vi "Bin2.vi"(11 "Image Src":T1) -> (3 "Image":T1(plugin-control))   [LabVIEW 2011]
uses:
  <vilib>/vision/Image Controls.llb/IMAQ Image.ctl
  <vilib>/vision/NI_Vision_Development_Module.lvlib
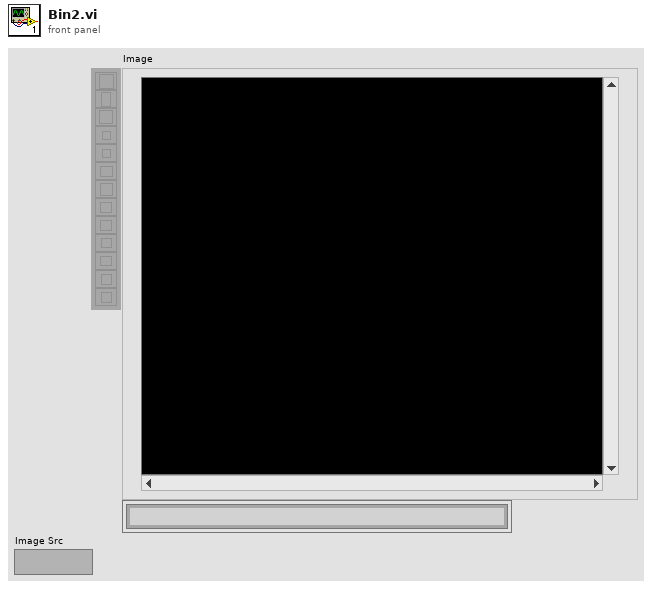
[diagram p1: front panel]
types:
  T1 = typedef "IMAQ Image.ctl" = refnum<image>
  T2 = typedef "Image Type" = u32
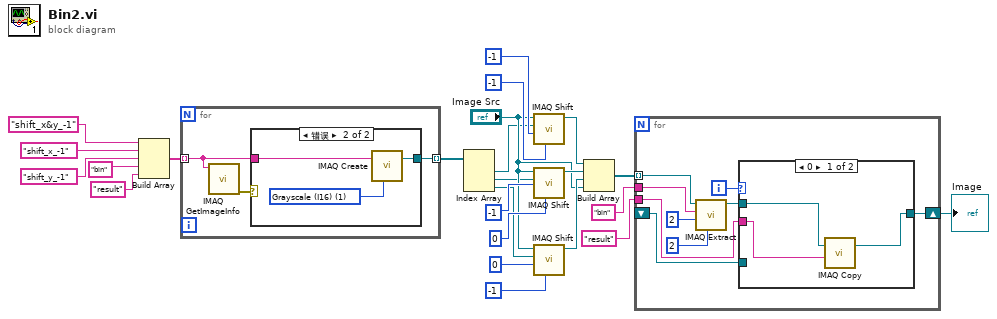
[diagram p0: block diagram]
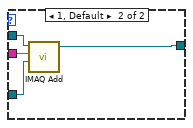
[diagram p3: hidden frame]
diagram:
  n1 = Build Array("shift_x&y_-1" ("Image Name"), "shift_x_-1" ("Image Name"), "shift_y_-1" ("Image Name"), "bin" ("Image Name"), "result" ("Image Name")) -> (w12:string[])
  n2 = for {
    tunnel: w12 -> [w26] mode=indexing
    tunnel: [w25] -> w8 mode=indexing
    n3 = call "IMAQ GetImageInfo"("Image"=w26) -> ("error out"=w27:errorcluster)  [unwired: 3 in, 7 out]
    n4 = case shown="错误" w27 {
      tunnel: w26 -> [w28 w30]
      tunnel: [w28 w29] -> w25
      frame No Error {
      }
      frame Error {
        w31 = T2 1 items=["Grayscale (U8)", "Grayscale (I16)", "Grayscale (SGL)", "Complex (CSG)", "RGB (U32)", "HSL (U32)", "RGB (U64)", "Grayscale (U16)"] ("Image Type")
        n5 = call "IMAQ Create"("Image Name"=w30, "Image Type"=w31) -> ("New Image"=w29:T1)  [unwired: 3 in, 1 out]
      }
    }
  }
  n6 = Index Array(array=w8) -> (element #1=w7:T1, element #2=w6:T1, element #3=w5:T1)  [unwired: 3 in]
  n7 = call "IMAQ Shift"("YOffset"=-1, "XOffset"=-1, "Image Dst"=w7, "Image Src"="Image Src") -> ("Image Dst Out"=w18:T1)  [unwired: 6 in, 1 out]
  n8 = call "IMAQ Shift"("YOffset"=0, "XOffset"=-1, "Image Dst"=w6, "Image Src"="Image Src") -> ("Image Dst Out"=w17:T1)  [unwired: 6 in, 1 out]
  n9 = call "IMAQ Shift"("YOffset"=-1, "XOffset"=0, "Image Dst"=w5, "Image Src"="Image Src") -> ("Image Dst Out"=w16:T1)  [unwired: 6 in, 1 out]
  n10 = Build Array(w18, w17, w16, "Image Src") -> (w15:T1[])
  n11 = for {
    tunnel: w15 -> [w37] mode=indexing
    shift-right: [w35] -> w14
    shift-left: _ -> [w34]
    tunnel: "bin" ("Image Name") -> [w33]
    tunnel: "result" ("Image Name") -> [w32]
    i -> [w40]
    n12 = call "IMAQ Extract"("Y Step Size"=2, "X Step Size"=2, "Image Dst"=w33, "Image Src"=w37) -> ("Image Dst Out"=w36:T1)  [unwired: 6 in, 1 out]
    n13 = case shown="0" w40 {
      tunnel: w36 -> [w43 w47]
      tunnel: [w41 w44] -> w35
      tunnel: w34 -> [_ w46]
      tunnel: w32 -> [w42 w45]
      frame 0 {
        n14 = call "IMAQ Copy"("Image Dst"=w42, "Image Src"=w43) -> ("Image Dst Out"=w41:T1)  [unwired: 4 in, 1 out]
      }
      frame 1, Default {
        n15 = call "IMAQ Add"("Image Src A"=w47, "Image Dst"=w45, "Image Src B"=w46) -> ("Image Dst Out"=w44:T1)  [unwired: 4 in, 1 out]
      }
    }
  }
  "Image" <- w14
